vi "氨氮启动命令.vi"(11 "参数":T1={"站号"=1, "量程切换"=enum."AUTO", "控制命令"=enum."启动测量", "模式设置"=enum."待机", "测量间隔"=0} {"站号" items=["总磷"=1, "总氮"=2, "氨氮"=3]}) -> (3 "启动命令":cluster{"命令":string, "data":variant})   [LabVIEW 2016, in "斯坦道氨氮.lvlib"]
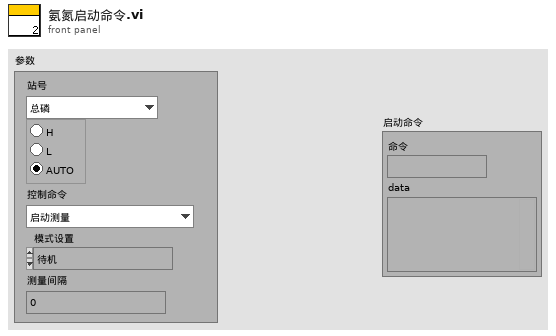
[diagram p1: front panel]
types:
  T1 = cluster{"站号":u16, "量程切换":enum32{"H", "L", "AUTO"}, "控制命令":enum16{"启动测量", "标样核查", "零点核查", "跨度核查", "空白测试", "平行样测试", "加标回收", "空白校准", "标样校准", "初始化（清洗）", "停止测试", "仪器重启", "校时", "模式设置", "测量间隔设置"}, "模式设置":enum16{"待机", "连续模式", "周期模式", "定点模式", "受控模式", "手动模式"}, "测量间隔":u16}
  T2 = enum16{"启动测量", "标样核查", "零点核查", "跨度核查", "空白测试", "平行样测试", "加标回收", "空白校准", "标样校准", "初始化（清洗）", "停止测试", "仪器重启", "校时", "模式设置", "测量间隔设置"}
  T3 = enum16{"待机", "连续模式", "周期模式", "定点模式", "受控模式", "手动模式"}
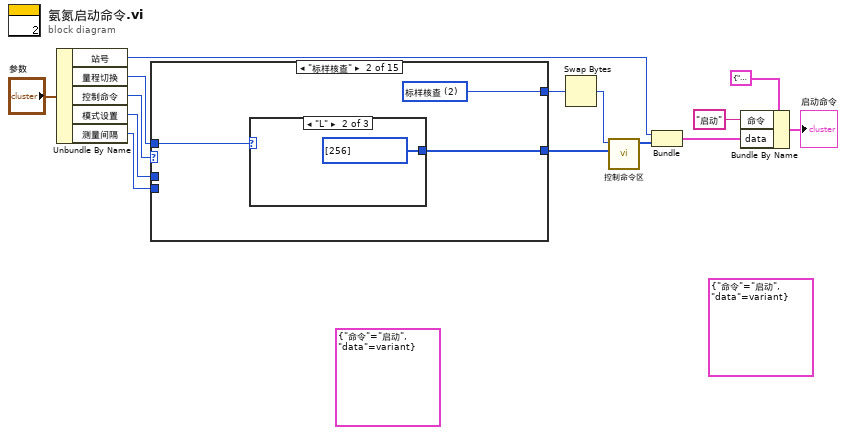
[diagram p0: block diagram]
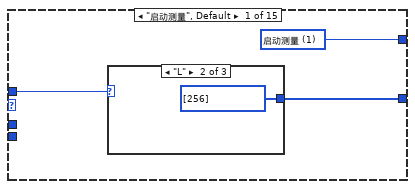
[diagram p2: hidden frame]
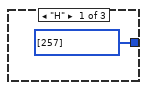
[diagram p3: hidden frame]
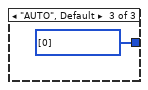
[diagram p4: hidden frame]
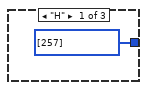
[diagram p5: hidden frame]
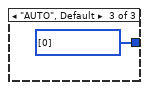
[diagram p6: hidden frame]
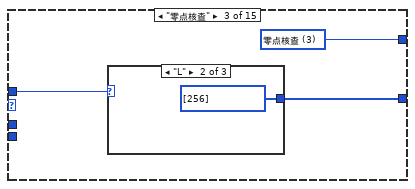
[diagram p7: hidden frame]
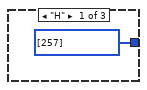
[diagram p8: hidden frame]
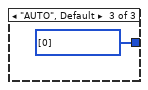
[diagram p9: hidden frame]
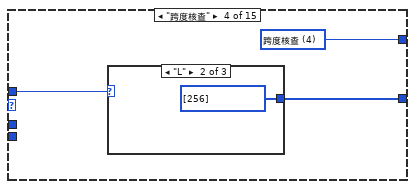
[diagram p10: hidden frame]
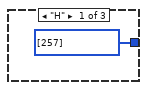
[diagram p11: hidden frame]
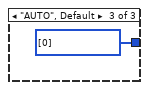
[diagram p12: hidden frame]
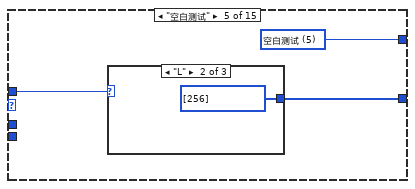
[diagram p13: hidden frame]
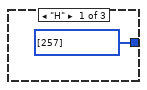
[diagram p14: hidden frame]
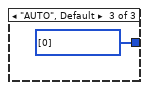
[diagram p15: hidden frame]
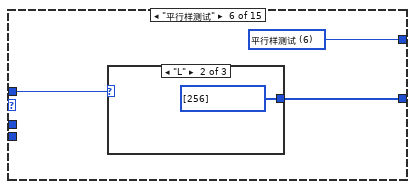
[diagram p16: hidden frame]
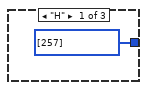
[diagram p17: hidden frame]
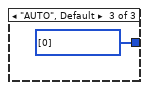
[diagram p18: hidden frame]
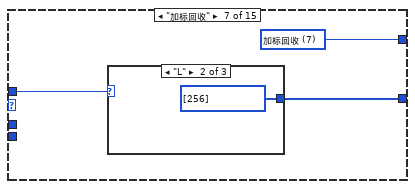
[diagram p19: hidden frame]
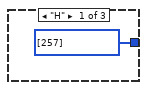
[diagram p20: hidden frame]
diagram:
  (unwired) cluster{"命令":string, "data":variant} {"命令"="启动", "data"=variant(cluster{"站号":u16, "控制命令":u16[]} {"站号"=3, "控制命令"=[2304, 0]})} ("启动命令")
  (unwired) cluster{"命令":string, "data":variant} {"命令"="启动", "data"=variant(cluster{"站号":u16, "控制命令":u16[]} {"站号"=3, "控制命令"=[2048, 0]})} ("启动命令")
  n1 = Unbundle By Name("参数") -> ("站号"=w12:u16, "量程切换"=w11:enum32{"H", "L", "AUTO"}, "控制命令"=w10:T2, "模式设置"=w8:T3, "测量间隔"=w9:u16)
  n2 = case shown="\"标样核查\"" w10 {
    tunnel: [w15 w21 w27 w33 w39 w45 w51 w57 w63 i32[] [] i32[] [] i32[] [] w75 w81 w91] -> w3
    tunnel: w11 -> [w17 w23 w29 w35 w41 w47 w53 w59 w65 _ _ _ _ _ _]
    tunnel: [w16 w22 w28 w34 w40 w46 w52 w58 w64 w69 w71 w73 w76 w83 w93] -> w2
    tunnel: w9 -> [_ _ _ _ _ _ _ _ _ _ _ _ _ _ w90]
    tunnel: w8 -> [_ _ _ _ _ _ _ _ _ _ _ _ _ w80 _]
    frame "启动测量", Default {
      w16 = u16 1 items=["启动测量"=1, "标样核查"=2, "零点核查"=3, "跨度核查"=4, "空白测试"=5, "平行样测试"=6, "加标回收"=7, "空白校准"=8, "标样校准"=9, "初始化（清洗）"=10, "停止测试"=11, "仪器重启"=12, "校时"=13, "模式设置"=14, "测量间隔设置"=15] ("控制命令")
      n3 = case shown="\"L\"" w17 {
        tunnel: [i32[] [257] i32[] [256] i32[] [0]] -> w15
        frame "H" {
        }
        frame "L" {
        }
        frame "AUTO", Default {
        }
      }
    }
    frame "标样核查" {
      w22 = u16 2 items=["启动测量"=1, "标样核查"=2, "零点核查"=3, "跨度核查"=4, "空白测试"=5, "平行样测试"=6, "加标回收"=7, "空白校准"=8, "标样校准"=9, "初始化（清洗）"=10, "停止测试"=11, "仪器重启"=12, "校时"=13, "模式设置"=14, "测量间隔设置"=15] ("控制命令")
      n4 = case shown="\"L\"" w23 {
        tunnel: [i32[] [257] i32[] [256] i32[] [0]] -> w21
        frame "H" {
        }
        frame "L" {
        }
        frame "AUTO", Default {
        }
      }
    }
    frame "零点核查" {
      w28 = u16 3 items=["启动测量"=1, "标样核查"=2, "零点核查"=3, "跨度核查"=4, "空白测试"=5, "平行样测试"=6, "加标回收"=7, "空白校准"=8, "标样校准"=9, "初始化（清洗）"=10, "停止测试"=11, "仪器重启"=12, "校时"=13, "模式设置"=14, "测量间隔设置"=15] ("控制命令")
      n5 = case shown="\"L\"" w29 {
        tunnel: [i32[] [257] i32[] [256] i32[] [0]] -> w27
        frame "H" {
        }
        frame "L" {
        }
        frame "AUTO", Default {
        }
      }
    }
    frame "跨度核查" {
      w34 = u16 4 items=["启动测量"=1, "标样核查"=2, "零点核查"=3, "跨度核查"=4, "空白测试"=5, "平行样测试"=6, "加标回收"=7, "空白校准"=8, "标样校准"=9, "初始化（清洗）"=10, "停止测试"=11, "仪器重启"=12, "校时"=13, "模式设置"=14, "测量间隔设置"=15] ("控制命令")
      n6 = case shown="\"L\"" w35 {
        tunnel: [i32[] [257] i32[] [256] i32[] [0]] -> w33
        frame "H" {
        }
        frame "L" {
        }
        frame "AUTO", Default {
        }
      }
    }
    frame "空白测试" {
      w40 = u16 5 items=["启动测量"=1, "标样核查"=2, "零点核查"=3, "跨度核查"=4, "空白测试"=5, "平行样测试"=6, "加标回收"=7, "空白校准"=8, "标样校准"=9, "初始化（清洗）"=10, "停止测试"=11, "仪器重启"=12, "校时"=13, "模式设置"=14, "测量间隔设置"=15] ("控制命令")
      n7 = case shown="\"L\"" w41 {
        tunnel: [i32[] [257] i32[] [256] i32[] [0]] -> w39
        frame "H" {
        }
        frame "L" {
        }
        frame "AUTO", Default {
        }
      }
    }
    frame "平行样测试" {
      w46 = u16 6 items=["启动测量"=1, "标样核查"=2, "零点核查"=3, "跨度核查"=4, "空白测试"=5, "平行样测试"=6, "加标回收"=7, "空白校准"=8, "标样校准"=9, "初始化（清洗）"=10, "停止测试"=11, "仪器重启"=12, "校时"=13, "模式设置"=14, "测量间隔设置"=15] ("控制命令")
      n8 = case shown="\"L\"" w47 {
        tunnel: [i32[] [257] i32[] [256] i32[] [0]] -> w45
        frame "H" {
        }
        frame "L" {
        }
        frame "AUTO", Default {
        }
      }
    }
    frame "加标回收" {
      w52 = u16 7 items=["启动测量"=1, "标样核查"=2, "零点核查"=3, "跨度核查"=4, "空白测试"=5, "平行样测试"=6, "加标回收"=7, "空白校准"=8, "标样校准"=9, "初始化（清洗）"=10, "停止测试"=11, "仪器重启"=12, "校时"=13, "模式设置"=14, "测量间隔设置"=15] ("控制命令")
      n9 = case shown="\"L\"" w53 {
        tunnel: [i32[] [257] i32[] [256] i32[] [0]] -> w51
        frame "H" {
        }
        frame "L" {
        }
        frame "AUTO", Default {
        }
      }
    }
    frame "空白校准" {
      w58 = u16 8 items=["启动测量"=1, "标样核查"=2, "零点核查"=3, "跨度核查"=4, "空白测试"=5, "平行样测试"=6, "加标回收"=7, "空白校准"=8, "标样校准"=9, "初始化（清洗）"=10, "停止测试"=11, "仪器重启"=12, "校时"=13, "模式设置"=14, "测量间隔设置"=15] ("控制命令")
      n10 = case shown="\"L\"" w59 {
        tunnel: [i32[] [257] i32[] [256] i32[] [0]] -> w57
        frame "H" {
        }
        frame "L" {
        }
        frame "AUTO", Default {
        }
      }
    }
    frame "标样校准" {
      w64 = u16 9 items=["启动测量"=1, "标样核查"=2, "零点核查"=3, "跨度核查"=4, "空白测试"=5, "平行样测试"=6, "加标回收"=7, "空白校准"=8, "标样校准"=9, "初始化（清洗）"=10, "停止测试"=11, "仪器重启"=12, "校时"=13, "模式设置"=14, "测量间隔设置"=15] ("控制命令")
      n11 = case shown="\"L\"" w65 {
        tunnel: [i32[] [257] i32[] [256] i32[] [0]] -> w63
        frame "H" {
        }
        frame "L" {
        }
        frame "AUTO", Default {
        }
      }
    }
    frame "初始化（清洗）" {
      w69 = u16 10 items=["启动测量"=1, "标样核查"=2, "零点核查"=3, "跨度核查"=4, "空白测试"=5, "平行样测试"=6, "加标回收"=7, "空白校准"=8, "标样校准"=9, "初始化（清洗）"=10, "停止测试"=11, "仪器重启"=12, "校时"=13, "模式设置"=14, "测量间隔设置"=15] ("控制命令")
    }
    frame "停止测试" {
      w71 = u16 11 items=["启动测量"=1, "标样核查"=2, "零点核查"=3, "跨度核查"=4, "空白测试"=5, "平行样测试"=6, "加标回收"=7, "空白校准"=8, "标样校准"=9, "初始化（清洗）"=10, "停止测试"=11, "仪器重启"=12, "校时"=13, "模式设置"=14, "测量间隔设置"=15] ("控制命令")
    }
    frame "仪器重启" {
      w73 = u16 12 items=["启动测量"=1, "标样核查"=2, "零点核查"=3, "跨度核查"=4, "空白测试"=5, "平行样测试"=6, "加标回收"=7, "空白校准"=8, "标样校准"=9, "初始化（清洗）"=10, "停止测试"=11, "仪器重启"=12, "校时"=13, "模式设置"=14, "测量间隔设置"=15] ("控制命令")
    }
    frame "校时" {
      w76 = u16 13 items=["启动测量"=1, "标样核查"=2, "零点核查"=3, "跨度核查"=4, "空白测试"=5, "平行样测试"=6, "加标回收"=7, "空白校准"=8, "标样校准"=9, "初始化（清洗）"=10, "停止测试"=11, "仪器重启"=12, "校时"=13, "模式设置"=14, "测量间隔设置"=15] ("控制命令")
      n12 = Get Date/Time In Seconds() -> (seconds since 1Jan1904=w79:timestamp)
      n13 = Insert Into Array(array=timestamp[] [] ("数组"), new element=w79) -> (w77:timestamp[])  [unwired: 1 in]
      n14 = call "DateToHex.vi"("DATE"=w77) -> ("数组"=w75:u16[])  [unwired: 10 in]
    }
    frame "模式设置" {
      w83 = u16 14 items=["启动测量"=1, "标样核查"=2, "零点核查"=3, "跨度核查"=4, "空白测试"=5, "平行样测试"=6, "加标回收"=7, "空白校准"=8, "标样校准"=9, "初始化（清洗）"=10, "停止测试"=11, "仪器重启"=12, "校时"=13, "模式设置"=14, "测量间隔设置"=15] ("控制命令")
      n15 = case shown="\"手动模式\"" w80 {
        tunnel: [i32[] [0] i32[] [1] i32[] [2] i32[] [3] i32[] [4] i32[] [5]] -> w82
        frame "待机", Default {
        }
        frame "连续模式" {
        }
        frame "周期模式" {
        }
        frame "定点模式" {
        }
        frame "受控模式" {
        }
        frame "手动模式" {
        }
      }
      n16 = call "HexToWord.vi"("数组"=w82) -> ("WORD"=w81:u16[])  [unwired: 10 in]
    }
    frame "测量间隔设置" {
      w93 = u16 15 items=["启动测量"=1, "标样核查"=2, "零点核查"=3, "跨度核查"=4, "空白测试"=5, "平行样测试"=6, "加标回收"=7, "空白校准"=8, "标样校准"=9, "初始化（清洗）"=10, "停止测试"=11, "仪器重启"=12, "校时"=13, "模式设置"=14, "测量间隔设置"=15] ("控制命令")
      n17 = Replace Array Subset(array=i32[] [0], new element=w90) -> (w92:i32[])  [unwired: 1 in]
      n18 = call "HexToWord.vi"("数组"=w92) -> ("WORD"=w91:u16[])  [unwired: 10 in]
    }
  }
  n19 = Swap Bytes(anything=w2) -> (byte swapped=w1:u16)
  n20 = call "控制命令区.vi"("控制命令参数"=w3, "控制命令"=w1) -> ("控制命令"=w7:u16[])  [unwired: 9 in]
  n21 = Bundle("站号"=w12, "控制命令"=w7) -> (w4:cluster{"站号":u16, "控制命令":u16[]})  [unwired: 1 in]
  n22 = Bundle By Name(cluster=cluster{"命令":string, "data":variant} {"命令"="", "data"=variant} ("元素"), "命令"="启动", "data"=w4) -> (→"启动命令":cluster{"命令":string, "data":variant})
